vi "SDO download (U16).vi"(6 "Value":u16, 7 "Wait?":bool, 8 "error in":errorcluster, 9 "Multiplexor":T1 {"Sub-Index" format="%.0x"; "Index" format="%04x"}, 10 "Node ID":u8, 11 "CANopen in":refnum<class "CANopen.lvclass">) -> (0 "error out":errorcluster, 3 "CANopen out":refnum<class "CANopen.lvclass">)   [LabVIEW 2026, in "canopen_.lvlib" / "CANopen.lvclass"]
doc: "Writes a value in the open dictionary of a CANopen node."
uses:
  CANopen.lvclass
  CANopen.lvclass/CANopen.ctl
  Multiplexor.ctl
  CANopen Master.lvlib
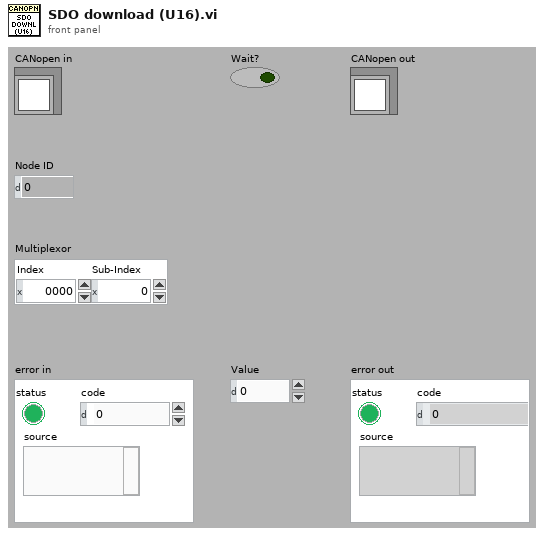
[diagram p1: front panel]
types:
  T1 = typedef "CANopen Master.lvlib/Multiplexor.ctl" = cluster{"Index":u16, "Sub-Index":i16}
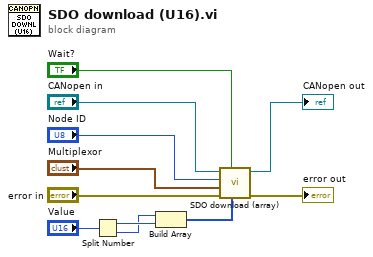
[diagram p0: block diagram]
diagram:
  n1 = Split Number(x="Value") -> (hi(x)=w4:u8, lo(x)=w3:u8)
  n2 = Build Array(w3, w4) -> (w5:u8[])
  n3 = call "SDO download (array).vi"("Value"=w5, "Wait?"="Wait?", "error in"="error in", "Multiplexor"="Multiplexor", "Node ID"="Node ID", "CANopen in"="CANopen in") -> ("error out"=→"error out":errorcluster, "CANopen out"=→"CANopen out":refnum<class "CANopen.lvclass">)  [unwired: 4 in]
